vi "Snd Play Wave File+.vi"(8 "error in (no error)":errorcluster, 10 "wait until finish (T)":bool=TRUE, 11 "wave file path in":path) -> (0 "error out":errorcluster, 3 "wave file path out":path)   [LabVIEW 2017]
doc: "Plays a sound file from disk. On the Macintosh operating system, AIFF and AIFF-C formats are supported and the VI returns immediately."
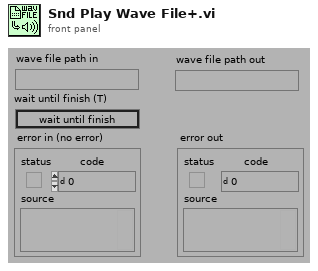
[diagram p1: front panel]
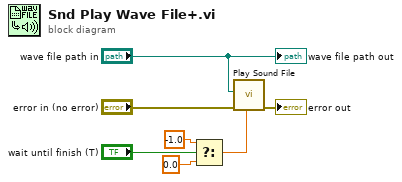
[diagram p0: block diagram]
diagram:
  n1 = Select(t=-1.0, s="wait until finish (T)", f=0.0 ("t")) -> (s? t:f=w1:dbl)
  n2 = call <vilib>:"Play Sound File.vi"("timeout (sec)"=w1, "error in (no error)"="error in (no error)", "path"="wave file path in") -> ("error out"=→"error out":errorcluster)  [unwired: 7 in, 1 out]
  "wave file path out" <- "wave file path in"
